vi "zmq_libpath.vi"() -> (0 "path":path)   [LabVIEW 2016, in "zeromq.lvlib"]
doc: "Returns an absolute path to the LVZMQ shared library on the host system."
uses:
  zeromq.lvlib
panel:
  # "ØMQ"
  # "labview"
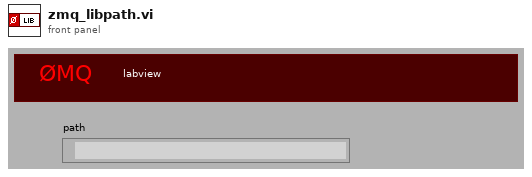
[diagram p1: front panel]
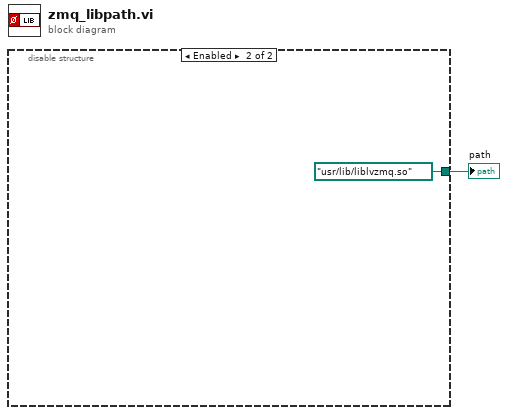
[diagram p0: block diagram]
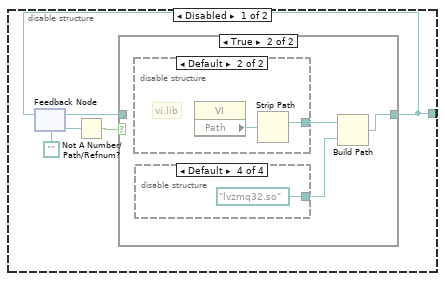
[diagram p2: hidden frame]
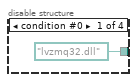
[diagram p4: hidden frame]
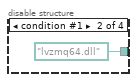
[diagram p5: hidden frame]
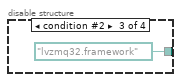
[diagram p6: hidden frame]
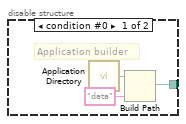
[diagram p7: hidden frame]
diagram:
  n1 = disable-structure shown="Enabled" {
    disable-tunnel: [w2 path "/usr/lib/liblvzmq.so" ("path")] -> w1
    frame Disabled {
      n2 = feedback #1(path "") -> (w3:path)
      n3 = Not A Number/Path/Refnum?(number/path/refnum=w3) -> (NaN/Path/Refnum?=w4:bool)
      n4 = case shown="True" w4 {
        tunnel: w3 -> [w6 _]
        tunnel: [w6 w7] -> w2
        frame False {
        }
        frame True {
          n5 = disable-structure shown="Default" {
            disable-tunnel: [w16 w18] -> w9
            frame condition #0 {
              # "Application builder"
              n6 = call <vilib>:"Application Directory.vi"() -> ("Application Directory"=w14:path)
              n7 = Build Path(base path=w14, name or relative path="data") -> (appended path=w16:path)
            }
            frame condition #1 (active) {
              # "vi.lib"
              n8 = property class="VI"() -> ("Path"=w17:path)  [unwired: 2 in, 2 out]
              n9 = Strip Path(path=w17) -> (stripped path=w18:path)  [unwired: 1 out]
            }
          }
          n10 = disable-structure shown="Default" {
            disable-tunnel: [path "lvzmq32.dll" ("appended path") path "lvzmq64.dll" ("appended path") path "lvzmq32.framework" ("appended path") path "lvzmq32.so" ("appended path")] -> w8
            frame condition #0 {
            }
            frame condition #1 {
            }
            frame condition #2 {
            }
            frame condition #3 (active) {
            }
          }
          n11 = Build Path(base path=w9, name or relative path=w8) -> (appended path=w7:path)
        }
      }
      n12 = feedback-in #1(w2) -> ()
    }
    frame Enabled {
    }
  }
  "path" <- w1
